vi "GUI_engineering_BACKUP_7Feb2011.vi"(4 "error in (no error)":errorcluster) -> (0 "error out":errorcluster, 2 "Canceled?":bool)   [LabVIEW 2015]
doc: "An editor for the motor manager parameters. Use this GUI to change the global variables assoicated with each motor. This VI does not write the changes to an engineering file."
uses:
  Systems/Slit/GSP_SLIT_Global.vi
  Systems/Grating_Translation/GSP_GT_Global.vi
  Systems/Primary Filter/GSP_F1_Global.vi
  Systems/Secondary Filter/GSP_F2_Global.vi
  GSCS Scripting/Utils/GSP_Wavelength_Global.vi
  Systems/Cam_Focus/GSP_CF_Global.vi
panel:
  in  "Undo":bool
  in  "Apply and Exit":bool
  in  "Tab Control":T1(tab)
  in  "GS Degrees at Home":dbl=20.4 caption="Degrees at home" format="%.2f"
  in  "GS Ticks per Degree":dbl=10000.0 caption="Ticks/degree" format="%.2f"
  in  "C - G min":dbl
  in  "C - G max":dbl
  in  "Grating min":dbl
  in  "Grating max":dbl=44.0
  in  "Camera min":dbl=-1.0
  in  "Camera max":dbl=88.0
  in  "Degrees at home":dbl=15.0 format="%.4f"
  in  "Ticks/degree":dbl=28571.43 format="%.4f"
  in  "F2 Offset to 1st Pos":i32 caption="Offset to 1st Pos"
  in  "F2 Counts per Position":dbl=6222.17 caption="Counts per Position" format="%.2f"
  in  "F1 Offset to 1st Pos":i32 caption="Offset to 1st Pos"
  in  "F1 Counts per Position":dbl=6222.17 caption="Counts per Position" format="%.2f"
  in  "Detent Position":i32
  in  "GT Offset to Clear Pos":i32=6580 caption="Offset to Clear Pos"
  in  "GT Offset between positions":i32=48715 caption="Offset Between Positions"
  in  "Offset to first Position":i32=175
  in  "Counts per Position":dbl=333.0 format="%.2f"
  in  "No Slit Position":i32=251743
  in  "Clear Position":i32=251743
  in  "Detent Position":i32=88865
  in  "Grab Position":i32=285543
  in  "Max Flex (deg)":dbl
  in  "B1 (microns)":dbl
  in  "Tilt (microns)":dbl
  in  "A2 (microns)":dbl
  in  "A1 (microns)":dbl
  # "Grating Stage"
  # "Interference (degrees)"
  # "Camera Stage"
  # "Secondary Wheel"
  # "Primary Wheel"
  # "Translation Stage"
  # "Translation Stage"
  # "Carousel"
  # "Camera offset = B1*(0.001/377.2)*\n\n(180/pi)*sin(rotator)"
  # "Camera stage"
  # "Left = -A1*cos(rotator)+(A2 + Tilt)*sin(rotator)+50\n\nRight = -A1*cos(rotator)+(A2 - Tilt)*sin(rotator)+50"
  # "Piezos"
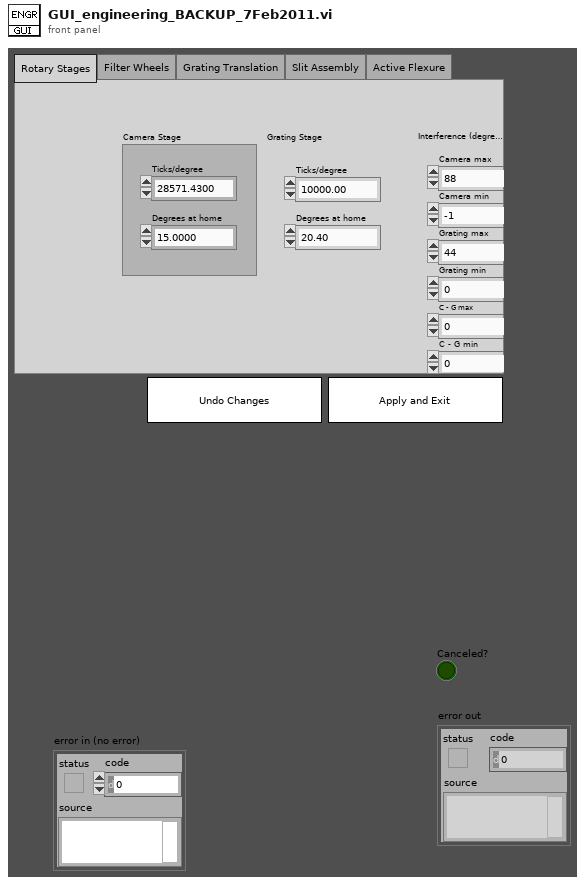
[diagram p1: front panel]
types:
  T1 = enum32{"Rotary Stages", "Filter Wheels", "Grating Translation", "Slit Assembly", "Active Flexure"}
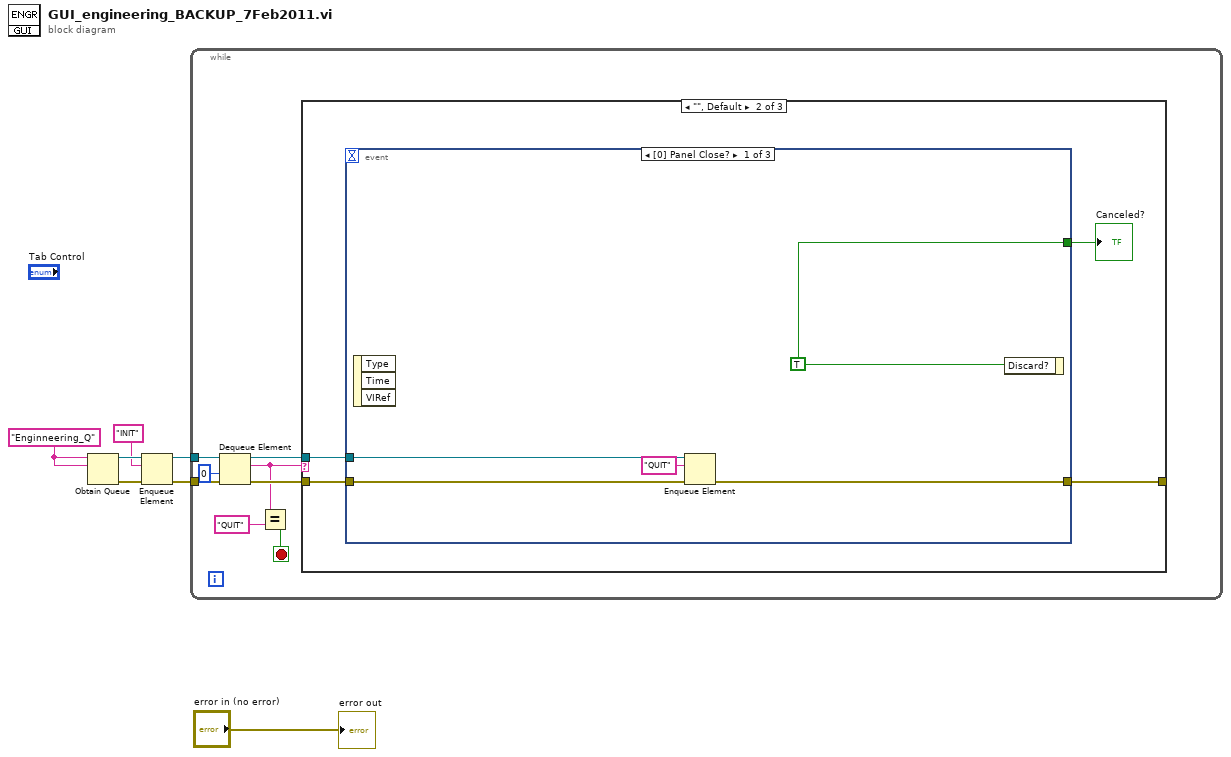
[diagram p0: block diagram]
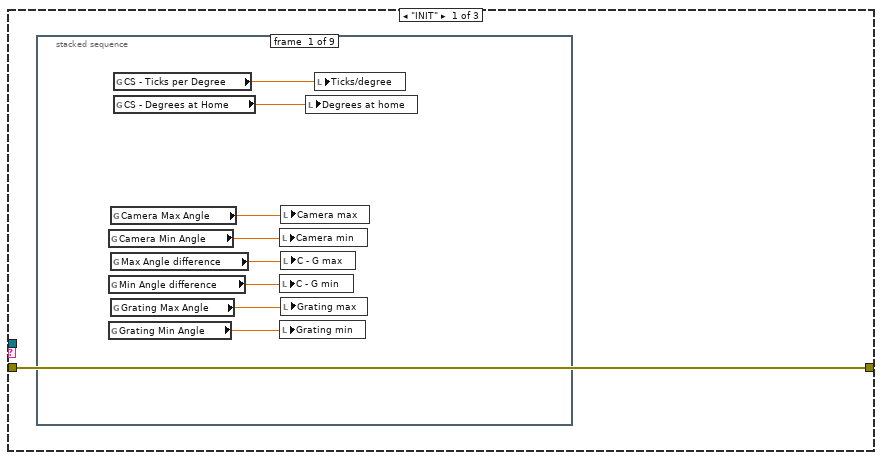
[diagram p2: hidden frame]
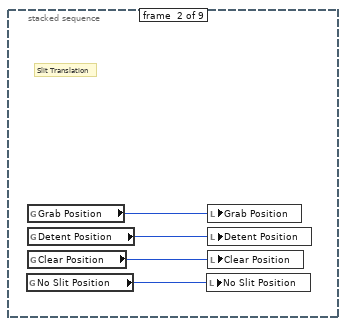
[diagram p3: hidden frame]
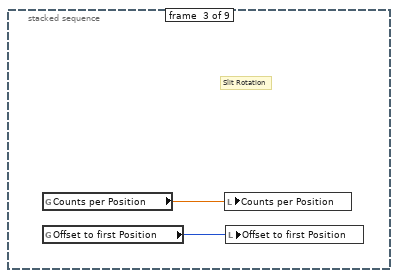
[diagram p4: hidden frame]
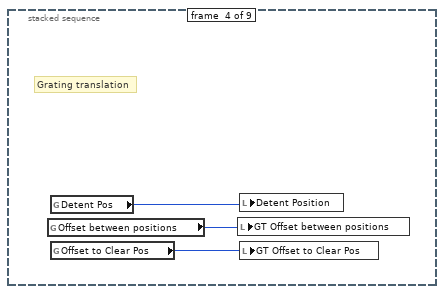
[diagram p5: hidden frame]
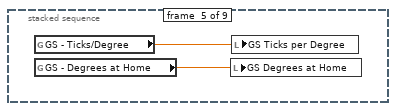
[diagram p6: hidden frame]
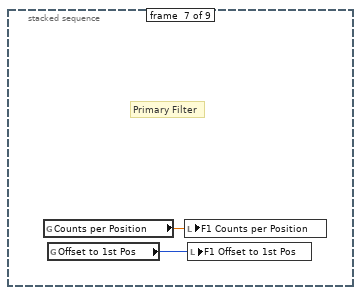
[diagram p8: hidden frame]
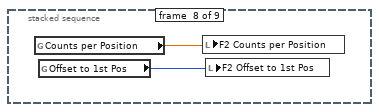
[diagram p9: hidden frame]
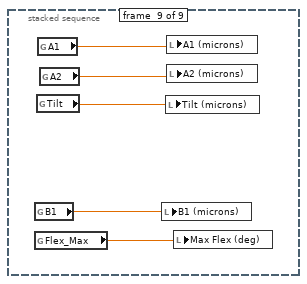
[diagram p10: hidden frame]
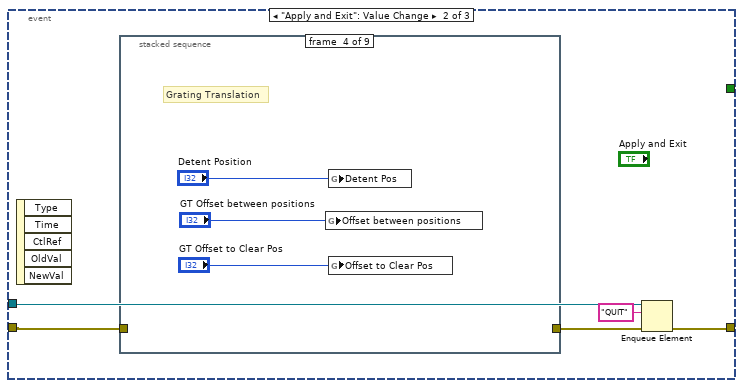
[diagram p11: hidden frame]
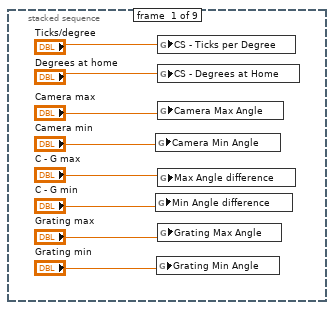
[diagram p12: hidden frame]
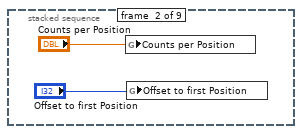
[diagram p13: hidden frame]
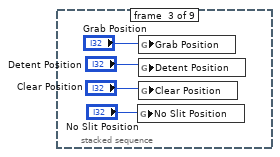
[diagram p14: hidden frame]
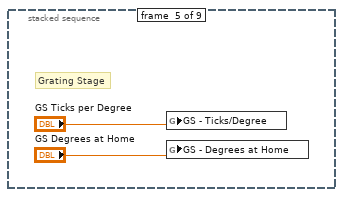
[diagram p15: hidden frame]
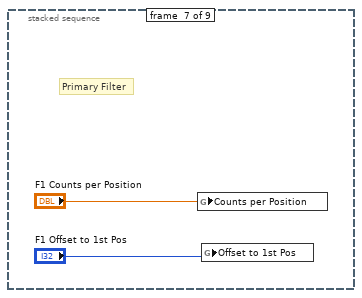
[diagram p17: hidden frame]
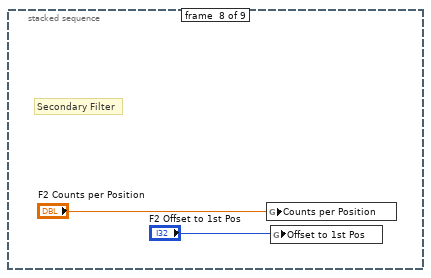
[diagram p18: hidden frame]
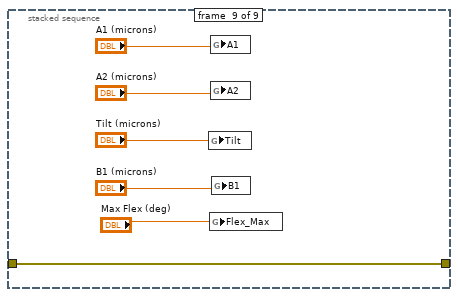
[diagram p19: hidden frame]
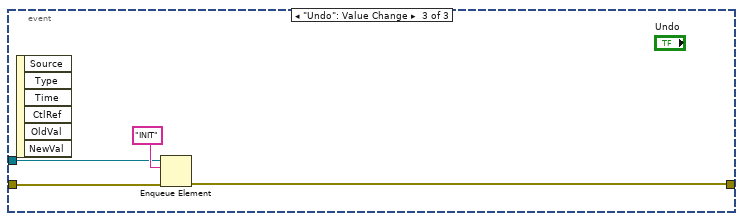
[diagram p20: hidden frame]
diagram:
  w3 = "Enginneering_Q"
  n1 = Obtain Queue(name (unnamed)=w3, element data type=w3) -> (queue out=w7:refnum<queue>, error out=w6:errorcluster)  [unwired: 3 in, 1 out]
  n2 = Enqueue Element(queue=w7, element="INIT", error in (no error)=w6) -> (queue out=w5:refnum<queue>, error out=w4:errorcluster)  [unwired: 1 in, 1 out]
  n3 = while {
    tunnel: w5 -> [w15]
    tunnel: w4 -> [w14]
    stop <- w9 stop-if-true
    n4 = Dequeue Element(queue=w15, timeout in ms (-1)=0, error in (no error)=w14) -> (queue out=w12:refnum<queue>, element=w11:string, error out=w13:errorcluster)  [unwired: 1 out]
    n5 = Equal?(x=w11, y="QUIT") -> (x = y?=w9:bool)
    n6 = case shown="\"\", Default" w11 {
      tunnel: w13 -> [w16 w48 w92]
      tunnel: w12 -> [_ w47 _]
      tunnel: [w16 w46 w92] -> _
      frame "INIT" {
        n7 = stacked-sequence {
          frame #0 {
            n8 = global read "GSP_Wavelength_Global.vi" "Camera Min Angle"() -> (w18:dbl)
            n9 = global read "GSP_Wavelength_Global.vi" "Min Angle difference"() -> (w20:dbl)
            n10 = global read "GSP_Wavelength_Global.vi" "Grating Min Angle"() -> (w22:dbl)
            n11 = global read "GSP_Wavelength_Global.vi" "Camera Max Angle"() -> (w17:dbl)
            n12 = global read "GSP_Wavelength_Global.vi" "Max Angle difference"() -> (w19:dbl)
            n13 = global read "GSP_Wavelength_Global.vi" "Grating Max Angle"() -> (w21:dbl)
            n14 = global read "GSP_Wavelength_Global.vi" "CS - Ticks per Degree"() -> (w24:dbl)
            n15 = global read "GSP_Wavelength_Global.vi" "CS - Degrees at Home"() -> (w23:dbl)
            n16 = local write "Camera min"(w18) -> ()
            n17 = local write "C - G min"(w20) -> ()
            n18 = local write "Grating min"(w22) -> ()
            n19 = local write "Camera max"(w17) -> ()
            n20 = local write "C - G max"(w19) -> ()
            n21 = local write "Grating max"(w21) -> ()
            n22 = local write "Degrees at home"(w23) -> ()
            n23 = local write "Ticks/degree"(w24) -> ()
          }
          frame #1 {
            # "Slit Translation"
            n24 = global read "GSP_SLIT_Global.vi" "No Slit Position"() -> (w25:i32)
            n25 = global read "GSP_SLIT_Global.vi" "Grab Position"() -> (w28:i32)
            n26 = global read "GSP_SLIT_Global.vi" "Detent Position"() -> (w27:i32)
            n27 = global read "GSP_SLIT_Global.vi" "Clear Position"() -> (w26:i32)
            n28 = local write "No Slit Position"(w25) -> ()
            n29 = local write "Grab Position"(w28) -> ()
            n30 = local write "Detent Position"(w27) -> ()
            n31 = local write "Clear Position"(w26) -> ()
          }
          frame #2 {
            # "Slit Rotation"
            n32 = global read "GSP_SLIT_Global.vi" "Counts per Position"() -> (w30:dbl)
            n33 = global read "GSP_SLIT_Global.vi" "Offset to first Position"() -> (w29:i32)
            n34 = local write "Counts per Position"(w30) -> ()
            n35 = local write "Offset to first Position"(w29) -> ()
          }
          frame #3 {
            # "Grating translation"
            n36 = global read "GSP_GT_Global.vi" "Offset between positions"() -> (w32:i32)
            n37 = global read "GSP_GT_Global.vi" "Detent Pos"() -> (w31:i32)
            n38 = global read "GSP_GT_Global.vi" "Offset to Clear Pos"() -> (w33:i32)
            n39 = local write "GT Offset between positions"(w32) -> ()
            n40 = local write "Detent Position"(w31) -> ()
            n41 = local write "GT Offset to Clear Pos"(w33) -> ()
          }
          frame #4 {
            n42 = global read "GSP_Wavelength_Global.vi" "GS - Ticks/Degree"() -> (w35:dbl)
            n43 = global read "GSP_Wavelength_Global.vi" "GS - Degrees at Home"() -> (w34:dbl)
            n44 = local write "GS Degrees at Home"(w34) -> ()
            n45 = local write "GS Ticks per Degree"(w35) -> ()
          }
          frame #5 {
          }
          frame #6 {
            # "Primary Filter"
            n46 = global read "GSP_F1_Global.vi" "Counts per Position"() -> (w37:dbl)
            n47 = global read "GSP_F1_Global.vi" "Offset to 1st Pos"() -> (w36:i32)
            n48 = local write "F1 Counts per Position"(w37) -> ()
            n49 = local write "F1 Offset to 1st Pos"(w36) -> ()
          }
          frame #7 {
            n50 = global read "GSP_F2_Global.vi" "Counts per Position"() -> (w38:dbl)
            n51 = global read "GSP_F2_Global.vi" "Offset to 1st Pos"() -> (w39:i32)
            n52 = local write "F2 Counts per Position"(w38) -> ()
            n53 = local write "F2 Offset to 1st Pos"(w39) -> ()
          }
          frame #8 {
            n54 = global read "GSP_Wavelength_Global.vi" "B1"() -> (w44:dbl)
            n55 = global read "GSP_Wavelength_Global.vi" "Flex_Max"() -> (w40:dbl)
            n56 = global read "GSP_CF_Global.vi" "Tilt"() -> (w41:dbl)
            n57 = global read "GSP_CF_Global.vi" "A1"() -> (w43:dbl)
            n58 = global read "GSP_CF_Global.vi" "A2"() -> (w42:dbl)
            n59 = local write "B1 (microns)"(w44) -> ()
            n60 = local write "Tilt (microns)"(w41) -> ()
            n61 = local write "A1 (microns)"(w43) -> ()
            n62 = local write "A2 (microns)"(w42) -> ()
            n63 = local write "Max Flex (deg)"(w40) -> ()
          }
        }
      }
      frame "", Default {
        n64 = event shown="[0] Panel Close?" {
          selector: _ -> [_ _ _]
          dyn-events: _ -> [_ _ _]
          timeout: _ -> [_ _ _]
          tunnel: w48 -> [w53 w55 w89]
          tunnel: w47 -> [w52 w57 w90]
          tunnel: [w50 w56 w88] -> w46
          tunnel: [w49 _ _] -> w45
          event Panel Close? {
            w49 = TRUE
            n65 = event-data() -> ()  [unwired: 1 in, 3 out]
            n66 = Enqueue Element(queue=w52, element="QUIT", error in (no error)=w53) -> (error out=w50:errorcluster)  [unwired: 1 in, 2 out]
            n67 = event-data("Discard?"=w49) -> ()  [unwired: 1 in, 1 out]
          }
          event "Apply and Exit": Value Change {
            n68 = event-data() -> ()  [unwired: 1 in, 5 out]
            n69 = stacked-sequence {
              tunnel: w55 -> [_ _ _ _ _ _ _ _ w87]
              tunnel: [_ _ _ _ _ _ _ _ w87] -> w54
              frame #0 {
                n70 = global write "GSP_Wavelength_Global.vi" "Camera Min Angle"("Camera min") -> ()
                n71 = global write "GSP_Wavelength_Global.vi" "Min Angle difference"("C - G min") -> ()
                n72 = global write "GSP_Wavelength_Global.vi" "Grating Min Angle"("Grating min") -> ()
                n73 = global write "GSP_Wavelength_Global.vi" "CS - Ticks per Degree"("Ticks/degree") -> ()
                n74 = global write "GSP_Wavelength_Global.vi" "CS - Degrees at Home"("Degrees at home") -> ()
                n75 = global write "GSP_Wavelength_Global.vi" "Camera Max Angle"("Camera max") -> ()
                n76 = global write "GSP_Wavelength_Global.vi" "Max Angle difference"("C - G max") -> ()
                n77 = global write "GSP_Wavelength_Global.vi" "Grating Max Angle"("Grating max") -> ()
              }
              frame #1 {
                n78 = global write "GSP_SLIT_Global.vi" "Counts per Position"("Counts per Position") -> ()
                n79 = global write "GSP_SLIT_Global.vi" "Offset to first Position"("Offset to first Position") -> ()
              }
              frame #2 {
                n80 = global write "GSP_SLIT_Global.vi" "No Slit Position"("No Slit Position") -> ()
                n81 = global write "GSP_SLIT_Global.vi" "Grab Position"("Grab Position") -> ()
                n82 = global write "GSP_SLIT_Global.vi" "Detent Position"("Detent Position") -> ()
                n83 = global write "GSP_SLIT_Global.vi" "Clear Position"("Clear Position") -> ()
              }
              frame #3 {
                # "Grating Translation"
                n84 = global write "GSP_GT_Global.vi" "Offset between positions"("GT Offset between positions") -> ()
                n85 = global write "GSP_GT_Global.vi" "Detent Pos"("Detent Position") -> ()
                n86 = global write "GSP_GT_Global.vi" "Offset to Clear Pos"("GT Offset to Clear Pos") -> ()
              }
              frame #4 {
                # "Grating Stage"
                n87 = global write "GSP_Wavelength_Global.vi" "GS - Ticks/Degree"("GS Ticks per Degree") -> ()
                n88 = global write "GSP_Wavelength_Global.vi" "GS - Degrees at Home"("GS Degrees at Home") -> ()
              }
              frame #5 {
                # "Coll Focus"
              }
              frame #6 {
                # "Primary Filter"
                n89 = global write "GSP_F1_Global.vi" "Counts per Position"("F1 Counts per Position") -> ()
                n90 = global write "GSP_F1_Global.vi" "Offset to 1st Pos"("F1 Offset to 1st Pos") -> ()
              }
              frame #7 {
                # "Secondary Filter"
                n91 = global write "GSP_F2_Global.vi" "Counts per Position"("F2 Counts per Position") -> ()
                n92 = global write "GSP_F2_Global.vi" "Offset to 1st Pos"("F2 Offset to 1st Pos") -> ()
              }
              frame #8 {
                n93 = global write "GSP_CF_Global.vi" "Tilt"("Tilt (microns)") -> ()
                n94 = global write "GSP_Wavelength_Global.vi" "Flex_Max"("Max Flex (deg)") -> ()
                n95 = global write "GSP_CF_Global.vi" "A1"("A1 (microns)") -> ()
                n96 = global write "GSP_CF_Global.vi" "A2"("A2 (microns)") -> ()
                n97 = global write "GSP_Wavelength_Global.vi" "B1"("B1 (microns)") -> ()
              }
            }
            n98 = Enqueue Element(queue=w57, element="QUIT", error in (no error)=w54) -> (error out=w56:errorcluster)  [unwired: 1 in, 2 out]
          }
          event "Undo": Value Change {
            n99 = event-data() -> ()  [unwired: 1 in, 6 out]
            n100 = Enqueue Element(queue=w90, element="INIT", error in (no error)=w89) -> (error out=w88:errorcluster)  [unwired: 1 in, 2 out]
          }
        }
        "Canceled?" <- w45
      }
      frame "QUIT" {
      }
    }
  }
  "error out" <- "error in (no error)"
